vi "Process.vi"(8 "error in (no error)":errorcluster, 10 "Pound in":refnum<class "Pound.lvclass">, 11 "Qbus in":refnum<class "Qbus.lvclass">) -> (0 "error out":errorcluster)   [LabVIEW 2017, in "Trigger.lvlib"]
doc: "The Trigger process evaluates the expressions that define when a data group enters and exits operating states. After determining the current operating state of the data goup, this process evaluates the file-collection expression for that state to determine whether to collect a file."
uses:
  <vilib>/addons/InsightCM/Devices/Shared/Common/Trigger/Trigger.lvlib
  <vilib>/addons/Qbus/Qbus.lvclass
  <vilib>/NI/Software Watchdog/Pound/Pound.lvclass
  <vilib>/addons/InsightCM/Devices/Shared/Common/Trigger/controls/config.ctl
  <vilib>/NI/Software Watchdog/Watchdog/Watchdog.lvclass
  <vilib>/addons/TraceLogger/TraceLogger.lvlib
  <vilib>/addons/InsightCM/Devices/Shared/Common/ServerComm/ServerComm.lvlib
  <vilib>/addons/InsightCM/Devices/Shared/Common/DataFlow/DataFlow.lvlib
  <vilib>/addons/InsightCM/Utilities/GlobalConfiguration/GlobalConfiguration.lvlib
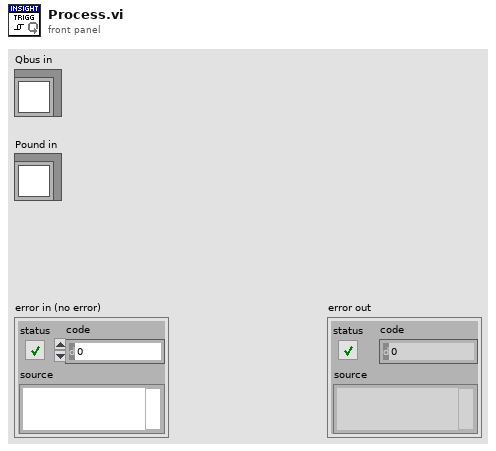
[diagram p1: front panel]
types:
  T1 = typedef "Trigger.lvlib/config.ctl" = cluster{"ForceTrig":variant, "OpStates":variant}
  T2 = typedef "DataFlow.lvlib/Data.ctl" = cluster{"DataGroup":string, "Waveforms":T3, "Map":T4, "Type":T5}
  T3 = typedef "wfmSGL_DVR.ctl" = refnum<data-value>
  T4 = typedef "PointValueMap.lvlib/PointMap.ctl" = refnum<data-value>
  T5 = typedef "DataFlow.lvlib/Type.ctl" = enum16{"High Rate", "Low Rate", "Burst Mode"}
  T6 = typedef "Message.ctl" = cluster{"Header":T7, "Body":u8[]}
  T7 = typedef "MessageHeader.ctl" = cluster{"MessageName":string, "Timestamp":i64, "CorrelationId":string, "ContentType":string, "RoutingKey":string, "Properties":T8[]}
  T8 = typedef "KeyValuePair.ctl" = cluster{"Key":string, "Value":string}
  T9 = typedef "DeviceForceTriggerRoutedMessageBody.ctl" = cluster{"DataGroup":string}
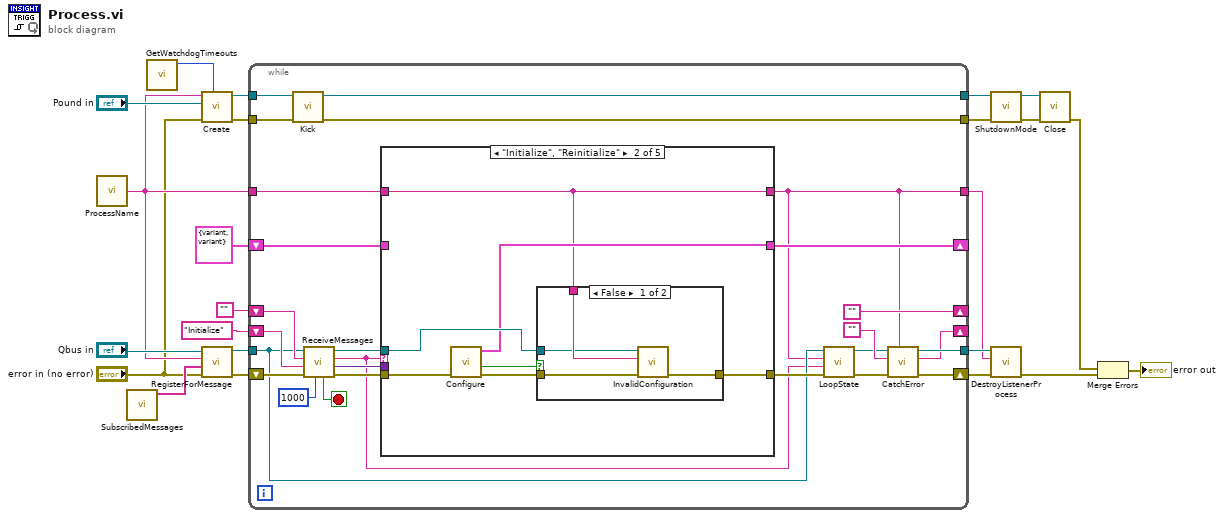
[diagram p0: block diagram]
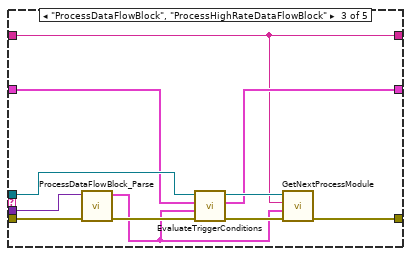
[diagram p4: hidden frame]
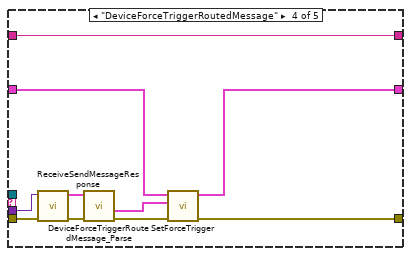
[diagram p5: hidden frame]
diagram:
  n1 = call <vilib>:"ProcessName.vi"() -> ("process name"=w11:string)  [unwired: 5 in]
  n2 = call <vilib>:"SubscribedMessages.vi"() -> ("subscribed messages"=w13:string[])  [unwired: 11 in]
  n3 = call <vilib>:"GetWatchdogTimeouts.vi"() -> ("software timeout"=w1:u32)  [unwired: 10 in, 1 out]
  n4 = call <vilib>:"Create.vi"("Execution Timeout (ms)"=w1, "error in (no error)"="error in (no error)", "Pound"="Pound in", "Name"=w11) -> ("error out"=w10:errorcluster, "Watchdog"=w9:refnum<data-value>)  [unwired: 6 in]
  n5 = call <vilib>:"RegisterForMessage.vi"("error in (no error)"="error in (no error)", "message names"=w13, "process name"=w11, "Qbus in"="Qbus in") -> ("error in (no error)"=w22:errorcluster, "Qbus out"=w21:refnum<class "Qbus.lvclass">)  [unwired: 6 in]
  n6 = while {
    shift-right: [""] -> _
    shift-left: "" -> [w47]
    tunnel: w21 -> [w33]
    tunnel: w11 -> [w35]
    tunnel: [w38] -> w18
    tunnel: [w28] -> w17
    shift-right: [w36] -> _
    shift-left: "Initialize" -> [w42]
    shift-right: [w40] -> _
    shift-left: T1 {"ForceTrig"=variant, "OpStates"=variant} ("config") -> [w41]
    tunnel: w10 -> [w32]
    tunnel: w9 -> [w31]
    tunnel: [w30] -> w5
    tunnel: [w29] -> w4
    shift-right: [w39] -> w20
    shift-left: w22 -> [w49]
    stop <- w48 stop-if-true
    n7 = call <vilib>:"Kick.vi"("error in (no error)"=w32, "Watchdog"=w31) -> ("error out"=w29:errorcluster, "Watchdog"=w30:refnum<data-value>)  [unwired: 8 in]
    n8 = call <vilib>:"ReceiveMessages.vi"("timeout (1000)"=1000 ("milliseconds to wait"), "error in (no error)"=w49, "priority action"=w42, "default action"=w47, "Qbus in"=w33) -> ("error out"=w46:errorcluster, "message value"=w43:variant, "action"=w27:string, "Qbus out"=w44:refnum<class "Qbus.lvclass">, "exit"=w48:bool)  [unwired: 2 in]
    n9 = case shown="\"Initialize\", \"Reinitialize\"" w27 {
      tunnel: w46 -> [w50 w57 w74 w80 w86]
      tunnel: w44 -> [_ w59 w68 _ _]
      tunnel: [w50 w58 w75 w82 w86] -> w34
      tunnel: w43 -> [_ _ w73 w79 _]
      tunnel: w41 -> [w52 _ w67 w84 w88]
      tunnel: [w52 w55 w71 w83 w88] -> w40
      tunnel: [w51 w54 w69 w85 w87] -> w28
      tunnel: w35 -> [w51 w54 w69 w85 w87]
      frame "", Default {
      }
      frame "Initialize", "Reinitialize" {
        n10 = call <vilib>:"Configure.vi"("error in (no error)"=w57) -> ("error out"=w56:errorcluster, "valid configuration"=w53:bool, "config"=w55:T1)  [unwired: 8 in]
        n11 = case shown="False" w53 {
          tunnel: w59 -> [w61 _]
          tunnel: [w63 w64] -> w58
          tunnel: w56 -> [w60 w64]
          tunnel: w54 -> [w62 _]
          frame False {
            n12 = call <vilib>:"InvalidConfiguration.vi"("error in (no error)"=w60, "description"=w62, "Qbus in"=w61) -> ("error out"=w63:errorcluster)  [unwired: 7 in, 1 out]
          }
          frame True {
          }
        }
      }
      frame "ProcessDataFlowBlock", "ProcessHighRateDataFlowBlock" {
        n13 = call <vilib>:"ProcessDataFlowBlock_Parse.vi"("error in (no error)"=w74, "body"=w73) -> ("error out"=w66:errorcluster, "data"=w65:T2)  [unwired: 8 in]
        n14 = call <vilib>:"EvaluateTriggerConditions.vi"("error in (no error)"=w66, "data"=w65, "config in"=w67, "Qbus in"=w68) -> ("error out"=w70:errorcluster, "config out"=w71:T1, "Qbus out"=w72:refnum<class "Qbus.lvclass">)  [unwired: 5 in]
        n15 = call <vilib>:"GetNextProcessModule.vi"("error in (no error)"=w70, "data"=w65, "source"=w69, "Qbus in"=w72) -> ("error out"=w75:errorcluster)  [unwired: 6 in, 1 out]
      }
      frame "DeviceForceTriggerRoutedMessage" {
        n16 = call <vilib>:"ReceiveSendMessageResponse.vi"("error in (no error)"=w80, "body"=w79) -> ("error out"=w78:errorcluster, "message"=w77:T6)  [unwired: 6 in, 2 out]
        n17 = call <vilib>:"DeviceForceTriggerRoutedMessage_Parse.vi"("error in (no error)"=w78, "Message"=w77) -> ("error out"=w81:errorcluster, "Body"=w76:T9)  [unwired: 6 in, 2 out]
        n18 = call <vilib>:"SetForceTrigger.vi"("error in (no error)"=w81, "body"=w76, "config in"=w84) -> ("error out"=w82:errorcluster, "config out"=w83:T1)  [unwired: 7 in]
      }
      frame "Exit" {
      }
    }
    n19 = call <vilib>:"LoopState.vi"("error in (no error)"=w34, "loop action"=w27, "process name"=w28, "Qbus in"=w33) -> ("error out"=w25:errorcluster, "Qbus out"=w24:refnum<class "Qbus.lvclass">)  [unwired: 6 in]
    n20 = call <vilib>:"CatchError.vi"("source"=w28, "error in (no error)"=w25, "next action in"="", "Qbus in"=w24) -> ("error out"=w39:errorcluster, "next action out"=w36:string, "Qbus out"=w38:refnum<class "Qbus.lvclass">)  [unwired: 5 in]
  }
  n21 = call <vilib>:"ShutdownMode.vi"("error in (no error)"=w4, "Watchdog"=w5) -> ("error out"=w7:errorcluster, "Watchdog"=w6:refnum<data-value>)  [unwired: 8 in]
  n22 = call <vilib>:"DestroyListenerProcess.vi"("error in (no error)"=w20, "process name"=w17, "Qbus in"=w18) -> ("error in (no error)"=w19:errorcluster)  [unwired: 7 in, 1 out]
  n23 = call <vilib>:"Close.vi"("error in (no error)"=w7, "Watchdog"=w6) -> ("error out"=w2:errorcluster)  [unwired: 9 in]
  n24 = Merge Errors(w2, w19) -> (→"error out":errorcluster)
